vi "SearchForApplications.vi"(8 "error in (no error)":errorcluster, 11 "MAUI.Editor in":refnum<class "MAUI.Editor.lvclass">) -> (0 "error out":errorcluster, 2 "folder names":string[](array[string]), 3 "MAUI.Editor out":refnum<class "MAUI.Editor.lvclass">)   [LabVIEW 2019, in "MAUI.Editor.lvclass"]
uses:
  MAUI.Editor.lvclass
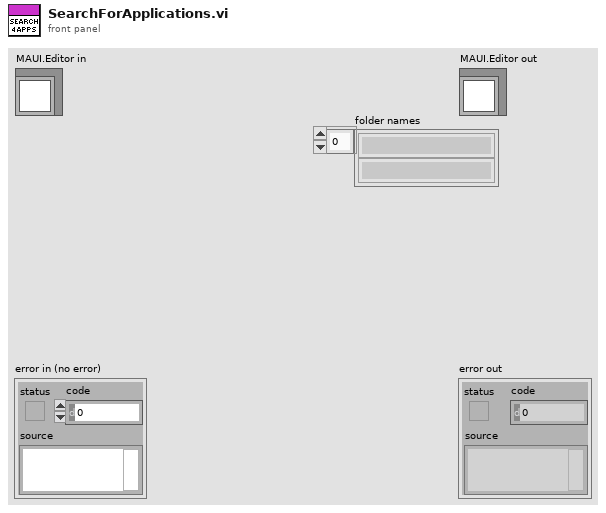
[diagram p1: front panel]
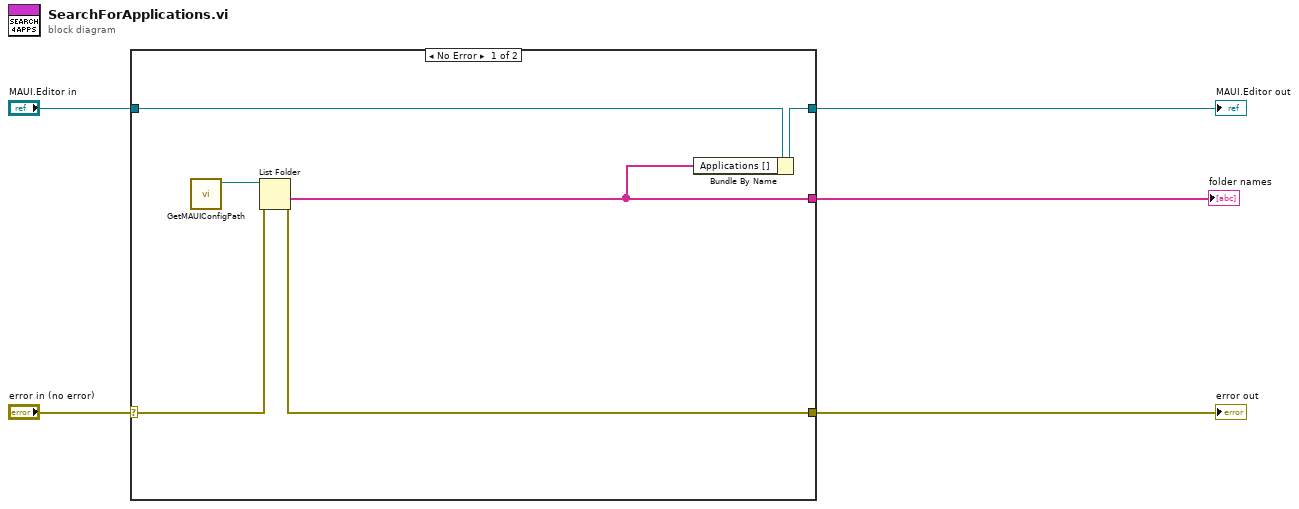
[diagram p0: block diagram]
diagram:
  n1 = case shown="No Error" "error in (no error)" {
    selector: "error in (no error)" -> [w10 w13]
    tunnel: [w9 w13] -> w4
    tunnel: [w8 w12] -> w2
    tunnel: "MAUI.Editor in" -> [w7 w12]
    tunnel: [w6 _] -> w1
    frame No Error {
      n2 = call "GetMAUIConfigPath.vi"() -> ("Default MAUI Path"=w11:path)  [unwired: 11 in]
      n3 = List Folder(path=w11, error in=w10) -> (folder names=w6:string[], error out=w9:errorcluster)  [unwired: 2 in, 2 out]
      n4 = Bundle By Name(cluster=w7, "Applications []"=w6) -> (w8:refnum<class "MAUI.Editor.lvclass">)
    }
    frame Error {
    }
  }
  "error out" <- w4
  "MAUI.Editor out" <- w2
  "folder names" <- w1
